vi "Is High Gear.vi"() -> ()   [LabVIEW 2017]
panel:
  out "High Gear?":bool
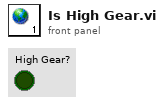
[diagram p1: front panel]
diagram:
